vi "SelectChildTag.vi"(10 "Name":string, 11 "ChildTag":string) -> (3 "Left Cell String":string)   [LabVIEW 2019, in "BlueVariantView.lvlib"]
uses:
  BlueVariantView.lvlib
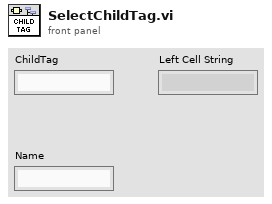
[diagram p1: front panel]
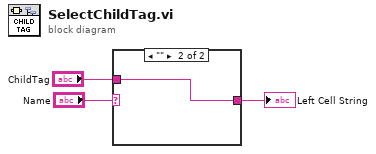
[diagram p0: block diagram]
diagram:
  n1 = case shown="\"\"" "Name" {
    selector: "Name" -> [w4 _]
    tunnel: [w4 w5] -> w2
    tunnel: "ChildTag" -> [_ w5]
    frame Default {
    }
    frame "" {
    }
  }
  "Left Cell String" <- w2
